vi "_S2P IMP Tree.vi"   [LabVIEW 2011]
uses:
  IMP Command.ctl
panel:
  # "See Diagram"
types:
  T1 = typedef "IMP Command.ctl" = enum16{"LOAD", "INITIALIZE", "IMPORT", "UNLOAD"}
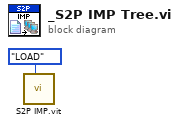
[diagram p0: block diagram]
diagram:
  n1 = call "S2P IMP.vit"("IMP Command"=IMP_Command."LOAD" ("VNA Command")) -> ()  [unwired: 2 in, 9 out]
